vi "AutoLin Protokoll CAL-Guete in StringArray.vi"(9 "MAN/AUTO":string, 10 "Sprachliste":string[][](array[string]), 11 "Lin-Polynom":T1 {"zusätzliche Zeitdauer Erster Punkt" format="%#_5g"; "Lin Modus" items=["Cal Gas to PNS", "Cal Gas to Samplepoint", "Measure"]; "Gas Ablaufdatum" format="%<%d.%m.%Y>T"; "HovaCAL Flow AutoLin"."HovaCAL Flow Input Cluster" format="%.2f"; "Gasflasche" items=["----"=10000, "IAG MG"=0, "IAG NH3 3000"=1, "IAG NH3 2000"=2, "IAG NH3 200"=3]; "Conditions:" items=["field", "laboratory"]; "Kalibrierauswahl" items=["Inaktiv", "Aktiv"]; "Anzahl Stufen" format="%#_5g"; "Zeitdauer Stufe" format="%#_5g"; "Verdünnungsgas" items=["N2", "O2"]; "Komponentenauswahl"."Konzentration" format="%#.6f"; "Gasnummer:" min=1 max=5; "Prüfgas Konzentration" format="%#.6f"; "Polynomkoeff." format="%#_18f"}) -> (3 "Lin-Güte (Protokoll)":string[][](array[string]))   [LabVIEW 2020, in "Linearisierung v2.lvlib" / "AutoLin Protokoll.lvlib"]
uses:
  AutoLin Protokoll.lvlib
  Lin-Polynom Daten.ctl
  KomponentenArray.ctl
  Visualisierungs Elemente/Auswahlfeld.ctl
  Visualisierungs Elemente/Zahlen-Eingabefeld.ctl
  EPA Optionsfeld.ctl
  Gasteiler/HovaCal/AutoLin Hovacal.ctl
  Kalibrieroption.ctl
  EPA1065-307/Condition.ctl
  Seiten/System Einstellungen V2/Konfig Gasflasche.ctl
  Seiten/System Einstellungen V2/Gasflasche Auswahl.ctl
  Gasteiler/HovaCAL_Interface/Controls/Flow Einstellung.ctl
  Gasteiler/HovaCAL_Interface/Controls/Pump state.ctl
  Seiten/CalGas Aufschaltung/Lin Modus.ctl
  Sprachverwaltung/Sprachverwaltung.lvlib
  Linearisierung v2.lvlib
  Gasteiler/Gasteiler.lvlib
  Gasteiler/HovaCal/HovaCal.lvlib
  EPA1065-307/Linearity verification 1065-307.lvlib
  Seiten/System Einstellungen V2/System Einstellungen V2.lvlib
  Gasteiler/HovaCAL_Interface/Controls/Controls.lvlib
  Seiten/CalGas Aufschaltung/CalGas Aufschaltung.lvlib
panel:
  # "%"
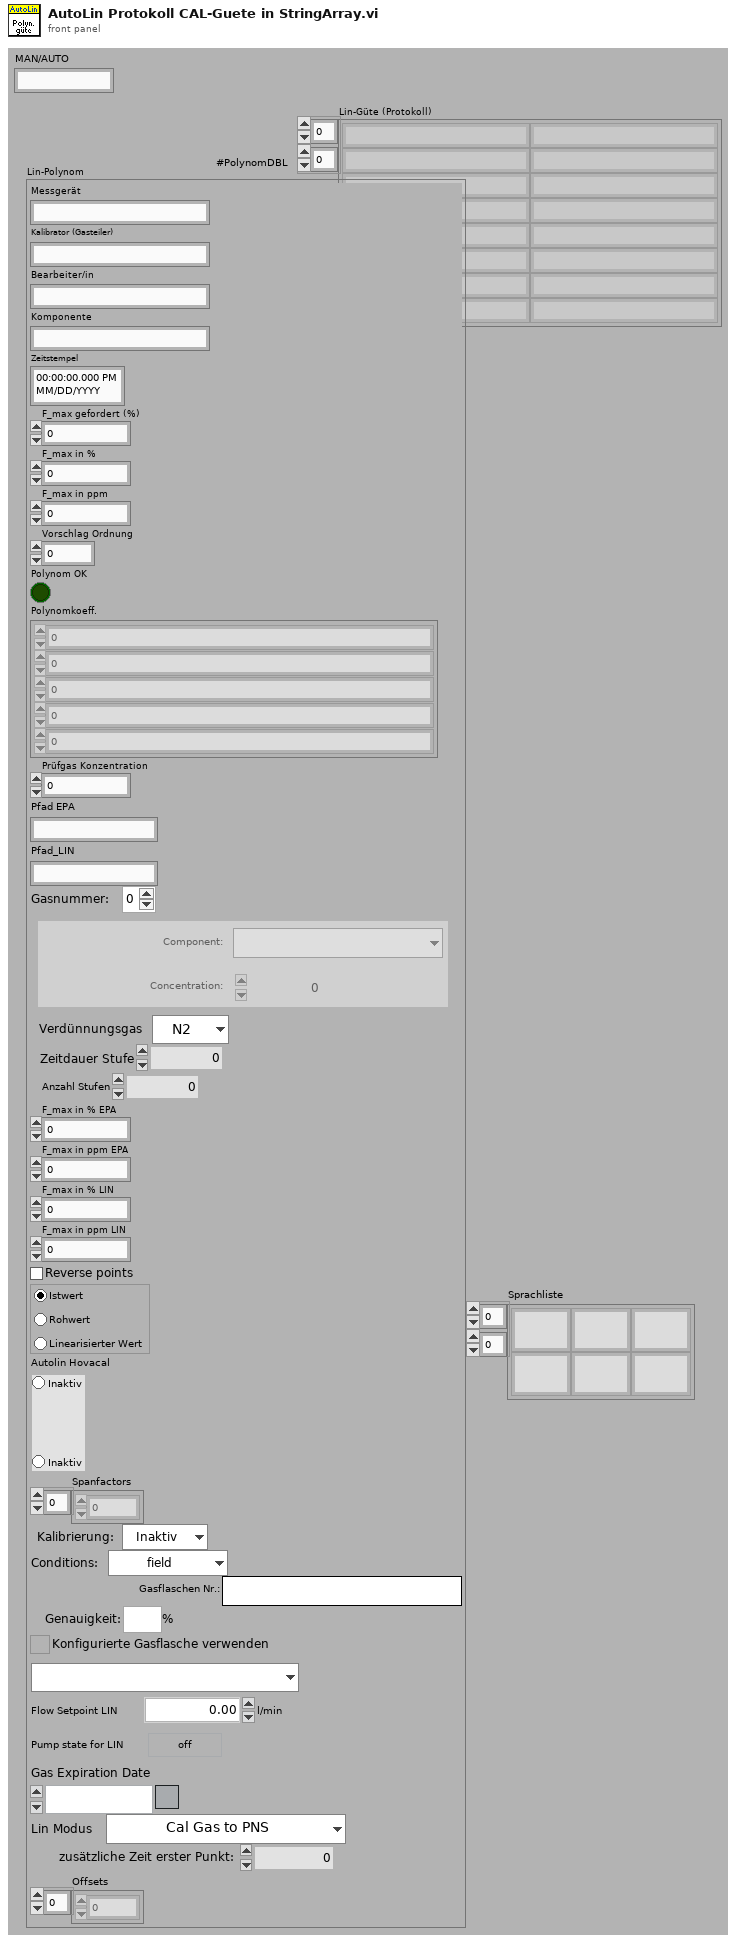
[diagram p1: front panel]
types:
  T1 = typedef "Linearisierung v2.lvlib/Lin-Polynom Daten.ctl" = cluster{"Messgerät":string, "Kalibrator (Gasteiler)":string, "Bearbeiter/in":string, "Komponente":string, "Zeitstempel":timestamp, "F_max gefordert (%)":sgl, "F_max in %":sgl, "F_max in ppm":sgl, "Vorschlag Ordnung":i32, "Polynom OK":bool, "Polynomkoeff.":dbl[], "Prüfgas Konzentration":dbl, "Pfad EPA":string, "Pfad_LIN":string, "Gasnummer:":u8, "Komponentenauswahl":T2, "Verdünnungsgas":T4, "Zeitdauer Stufe":T5, "Anzahl Stufen":T5, "F_max in % EPA":sgl, "F_max in ppm EPA":sgl, "F_max in % LIN":sgl, "F_max in ppm LIN":sgl, "Punkte umkehren":bool, "EPA Optionsfeld":T6, "Autolin Hovacal":T7, "Spanfactors":sgl[], "Kalibrierauswahl":T8, "Conditions:":T9, "Gasflaschen Nr.:":string, "Bottle Accuracy":dbl, "Konfig Gasflasche":T10, "Gasflasche":T11, "HovaCAL Flow AutoLin":T12, "MFC Output":T13, "Gas Ablaufdatum":timestamp, "Lin Modus":T14, "zusätzliche Zeitdauer Erster Punkt":sgl, "Offsets":sgl[]}
  T2 = typedef "Linearisierung v2.lvlib/KomponentenArray.ctl" = cluster{"Komponente:":T3, "Konzentration":dbl}[]
  T3 = typedef "Auswahlfeld.ctl" = u16
  T4 = typedef "Linearisierung v2.lvlib/Gasteiler.lvlib/Prüfgas in.ctl" = u16
  T5 = typedef "Zahlen-Eingabefeld.ctl" = sgl
  T6 = typedef "Linearisierung v2.lvlib/EPA Optionsfeld.ctl" = enum32{"Istwert", "Rohwert", "Linearisierter Wert"}
  T7 = typedef "Linearisierung v2.lvlib/Gasteiler.lvlib/HovaCal.lvlib/AutoLin Hovacal.ctl" = enum32{"Keine Auswahl", "Optionsauswahl 1", "Optionsauswahl 2"}
  T8 = typedef "Linearisierung v2.lvlib/Kalibrieroption.ctl" = u16
  T9 = typedef "Linearisierung v2.lvlib/Linearity verification 1065-307.lvlib/Condition.ctl" = u16
  T10 = typedef "System Einstellungen V2.lvlib/Konfig Gasflasche.ctl" = bool
  T11 = typedef "System Einstellungen V2.lvlib/Gasflasche Auswahl.ctl" = u16
  T12 = typedef "Linearisierung v2.lvlib/Gasteiler.lvlib/HovaCAL_Interface.lvlib/Controls.lvlib/Flow Einstellung.ctl" = cluster{"HovaCAL Flow Input Cluster":dbl}
  T13 = typedef "Linearisierung v2.lvlib/Gasteiler.lvlib/HovaCAL_Interface.lvlib/Controls.lvlib/Pump state.ctl" = cluster{"Run":bool}
  T14 = typedef "CalGas Aufschaltung.lvlib/Lin Modus.ctl" = u16
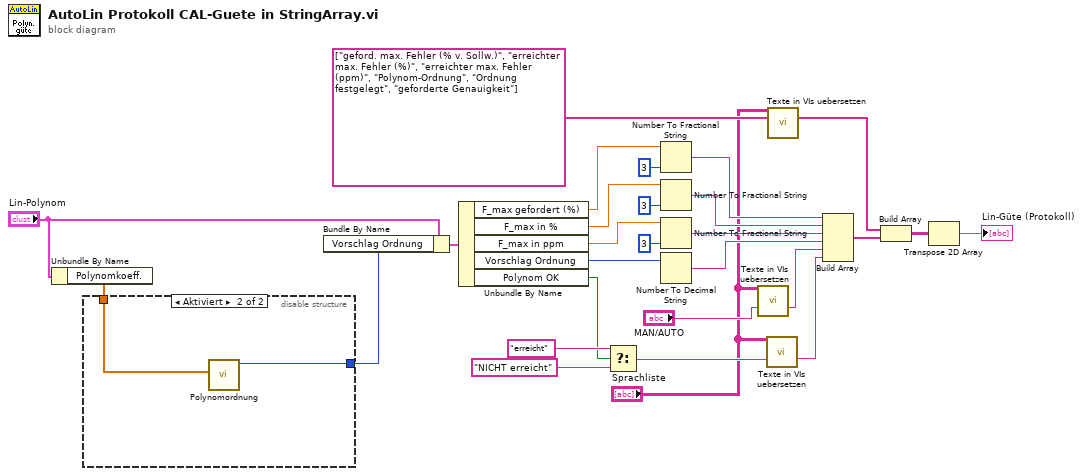
[diagram p0: block diagram]
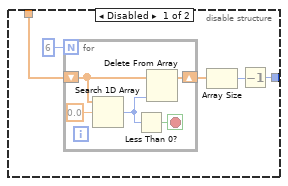
[diagram p2: hidden frame]
diagram:
  n1 = Unbundle By Name("Lin-Polynom") -> ("Polynomkoeff."=w9:dbl[])
  n2 = disable-structure shown="Aktiviert" {
    disable-tunnel: w9 -> [w33 w40]
    disable-tunnel: [w29 w39] -> w2
    frame Disabled {
      n3 = for {
        N: 6 -> [_]
        shift-right: [w36] -> w32
        shift-left: w33 -> [w37]
        stop <- w35 stop-if-true
        n4 = Search 1D Array(1D array=w37, element=sgl 0.0 ("Element")) -> (index of element=w34:i32)  [unwired: 1 in]
        n5 = Less Than 0?(x=w34) -> (x < 0?=w35:bool)
        n6 = Delete From Array(array=w37, index=w34) -> (array with subset deleted=w36:dbl[])  [unwired: 1 in, 1 out]
      }
      n7 = Array Size(array=w32) -> (size(s)=w30:i32)
      n8 = Decrement(x=w30) -> (x-1=w29:i32)
    }
    frame Enabled {
      n9 = call "Polynomordnung.vi"("LIN Polynom"=w40) -> ("Polynomordnung"=w39:i32)  [unwired: 9 in, 1 out]
    }
  }
  n10 = Bundle By Name(cluster="Lin-Polynom", "Vorschlag Ordnung"=w2) -> (w13:T1)
  n11 = Unbundle By Name(w13) -> ("F_max gefordert (%)"=w20:sgl, "F_max in %"=w21:sgl, "F_max in ppm"=w22:sgl, "Vorschlag Ordnung"=w12:i32, "Polynom OK"=w11:bool)
  n12 = Select(t="erreicht", s=w11, f="NICHT erreicht") -> (s? t:f=w8:string)
  n13 = Number To Fractional String(number=w20, precision (6)=i16 3 ("Genauigkeit (6)")) -> (F-format string=w25:string)  [unwired: 2 in]
  n14 = Number To Fractional String(number=w21, precision (6)=i16 3 ("Genauigkeit (6)")) -> (F-format string=w16:string)  [unwired: 2 in]
  n15 = Number To Fractional String(number=w22, precision (6)=i16 3 ("Genauigkeit (6)")) -> (F-format string=w26:string)  [unwired: 2 in]
  n16 = Number To Decimal String(number=w12) -> (decimal integer string=w10:string)  [unwired: 1 in]
  n17 = call "Texte in VIs uebersetzen.vi"("Sprachliste"="Sprachliste", "String zum Übersetzen"="MAN/AUTO") -> ("String zum Übersetzen"=w6:string)  [unwired: 9 in, 4 out]
  n18 = call "Texte in VIs uebersetzen.vi"("Sprachliste"="Sprachliste", "String zum Übersetzen"=w8) -> ("String zum Übersetzen"=w7:string)  [unwired: 9 in, 4 out]
  n19 = call "Texte in VIs uebersetzen.vi"("Sprachliste"="Sprachliste", "String-Array zum Übersetzen"=string[] ["geford. max. Fehler (% v. Sollw.)", "erreichter max. Fehler (%)", "erreichter max. Fehler (ppm)", "Polynom-Ordnung", "Ordnung festgelegt", "geforderte Genauigkeit"]) -> ("String-Array zum Übersetzen"=w4:string[])  [unwired: 9 in, 4 out]
  n20 = Build Array(w25, w16, w26, w10, w6, w7) -> (w19:string[])
  n21 = Build Array(w4, w19) -> (w18:string[][])
  n22 = Transpose 2D Array(2D array=w18) -> (transposed array=→"Lin-Güte (Protokoll)":string[][])
